vi "PID_2Chan_V3_multiple_avgs.vi"() -> ()   [LabVIEW 2016]
uses:
  <vilib>/addons/control/pid/pid.llb/PID Advanced (DBL Array).vi
  <vilib>/addons/control/pid/pid.llb/PID Parameter Manager (DBL Array).vi
  <vilib>/addons/control/pid/pid.llb/PID Derivative Action Buffered (DBL Array).vi
  <vilib>/addons/control/pid/pid.llb/PID Get Advanced Error (DBL Array).vi
  <vilib>/addons/control/pid/pid.llb/PID Integral Action Buffered (DBL Array).vi
  <vilib>/addons/control/pid/pid.llb/PID Resize 1D Array.vi
  <vilib>/addons/control/pid/pid.llb/PID Get Advanced Error (DBL).vi
  <userlib>/Fluigent/Fluigent MFCS/FluigentMFCS_Full.llb/MFCS_EZ Detect.vi
  <userlib>/Fluigent/Fluigent MFCS/FluigentMFCS_Full.llb/MFCS_EZ Initialization.vi
  <userlib>/Fluigent/Fluigent MFCS/FluigentMFCS_Full.llb/MFCS_EZ Write Channel Pressure.vi
  <userlib>/Fluigent/Fluigent MFCS/FluigentMFCS_Full.llb/MFCS_EZ Close.vi
  <vilib>/addons/control/pid/NI_PID_pid.lvlib
  <vilib>/Analysis/NI_AALBase.lvlib
  <vilib>/Analysis/baseanly.llb/Mean (DBL).vi
panel:
  in  "Vals to display":dbl=400.0
  out "F1 plot":dbl(graph)
  out "F tot":dbl
  in  "F2 PID gains":cluster{"P":dbl, "I":dbl, "D":dbl}={"P"=1.0, "I"=0.01, "D"=0.0} {"D" format="%.3f"; "I" format="%.3f"; "P" format="%.3f"}
  out "F1 Err":T1(graph)
  out "Pressures":dbl[](array[numeric])
  in  "F1 PID gains":cluster{"P":dbl, "I":dbl, "D":dbl}={"P"=1.0, "I"=0.01, "D"=0.0} {"D" format="%.3f"; "I" format="%.3f"; "P" format="%.3f"}
  in  "reinitialize? (F) 2":bool
  out "Flow 1":dbl
  in  "reset Averging":bool
  in  "Set current Pressure\n to manual pressure":bool
  out "Pressures":cluster{"[0]":dbl, "[1]":dbl}(graph)={"[0]"=667.158203125, "[1]"=642.5421752929688}
  out "F0 Err":T1(graph)
  in  "stop":bool=TRUE
  out "F total plot":dbl(graph)
  in  "Valves":enum16{"1", "2", "3", "4", "5", "6", "7", "8"}[](array[ring])=[enum."6", enum."7"]
  in  "Pressure Channels":i16[](array[numeric])=[2, 3]
  in  "Manual Pressure Set":dbl[](array[numeric])=[581.6619074041193, 548.1519459117543]
  in  "PID On":bool=TRUE
  in  "reinitialize? (F)":bool
  in  "Ftot Setpoint":dbl=350.0
  in  "F1 Setpoint":dbl=210.0
  in  "Add Ctrl?":bool
  in  "Boards":enum16{"A", "B", "C"}[](array[ring])=[enum."A", enum."A"]
  in  "Valves":enum16{"1", "2", "3", "4", "5", "6", "7", "8"}[](array[ring])=[enum."5", enum."4"]
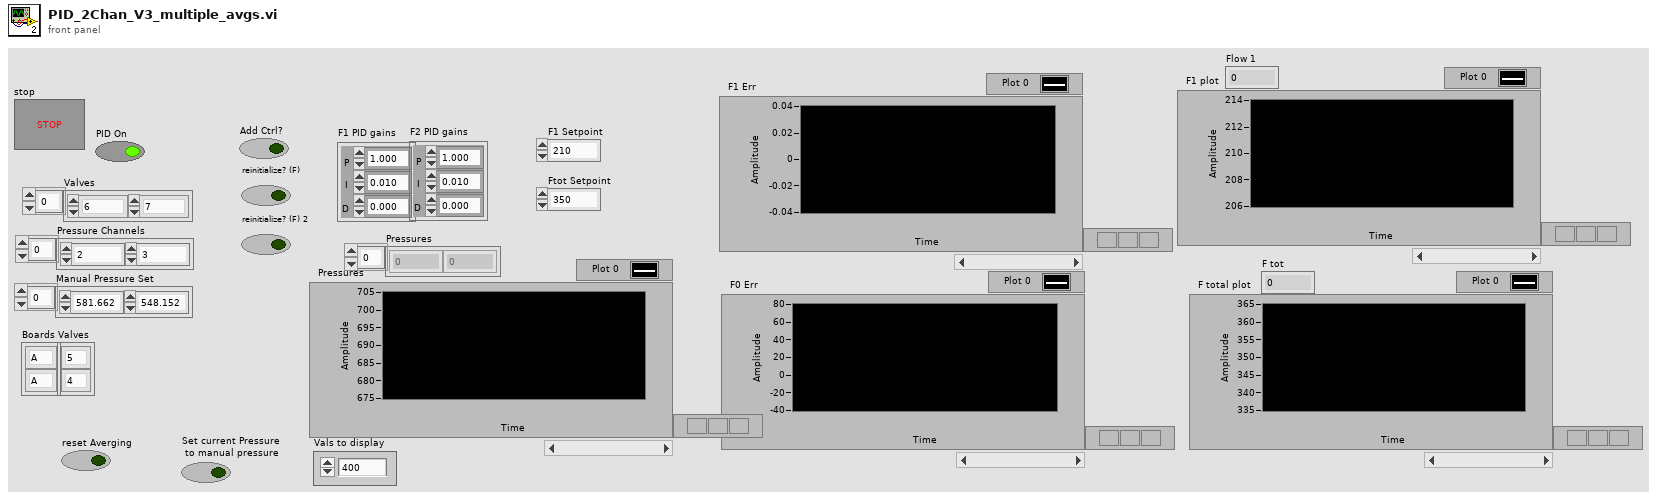
[diagram p1: front panel]
types:
  T1 = cluster{"output[0]":dbl, "output[1]":dbl, "output[2]":dbl}
  T2 = cluster{"setpoint high":dbl, "setpoint low":dbl}[]
  T3 = typedef "_EZmfcsSN.ctl" = u16
  T4 = typedef "_EZmfcsRefNum.ctl" = refnum<k1>
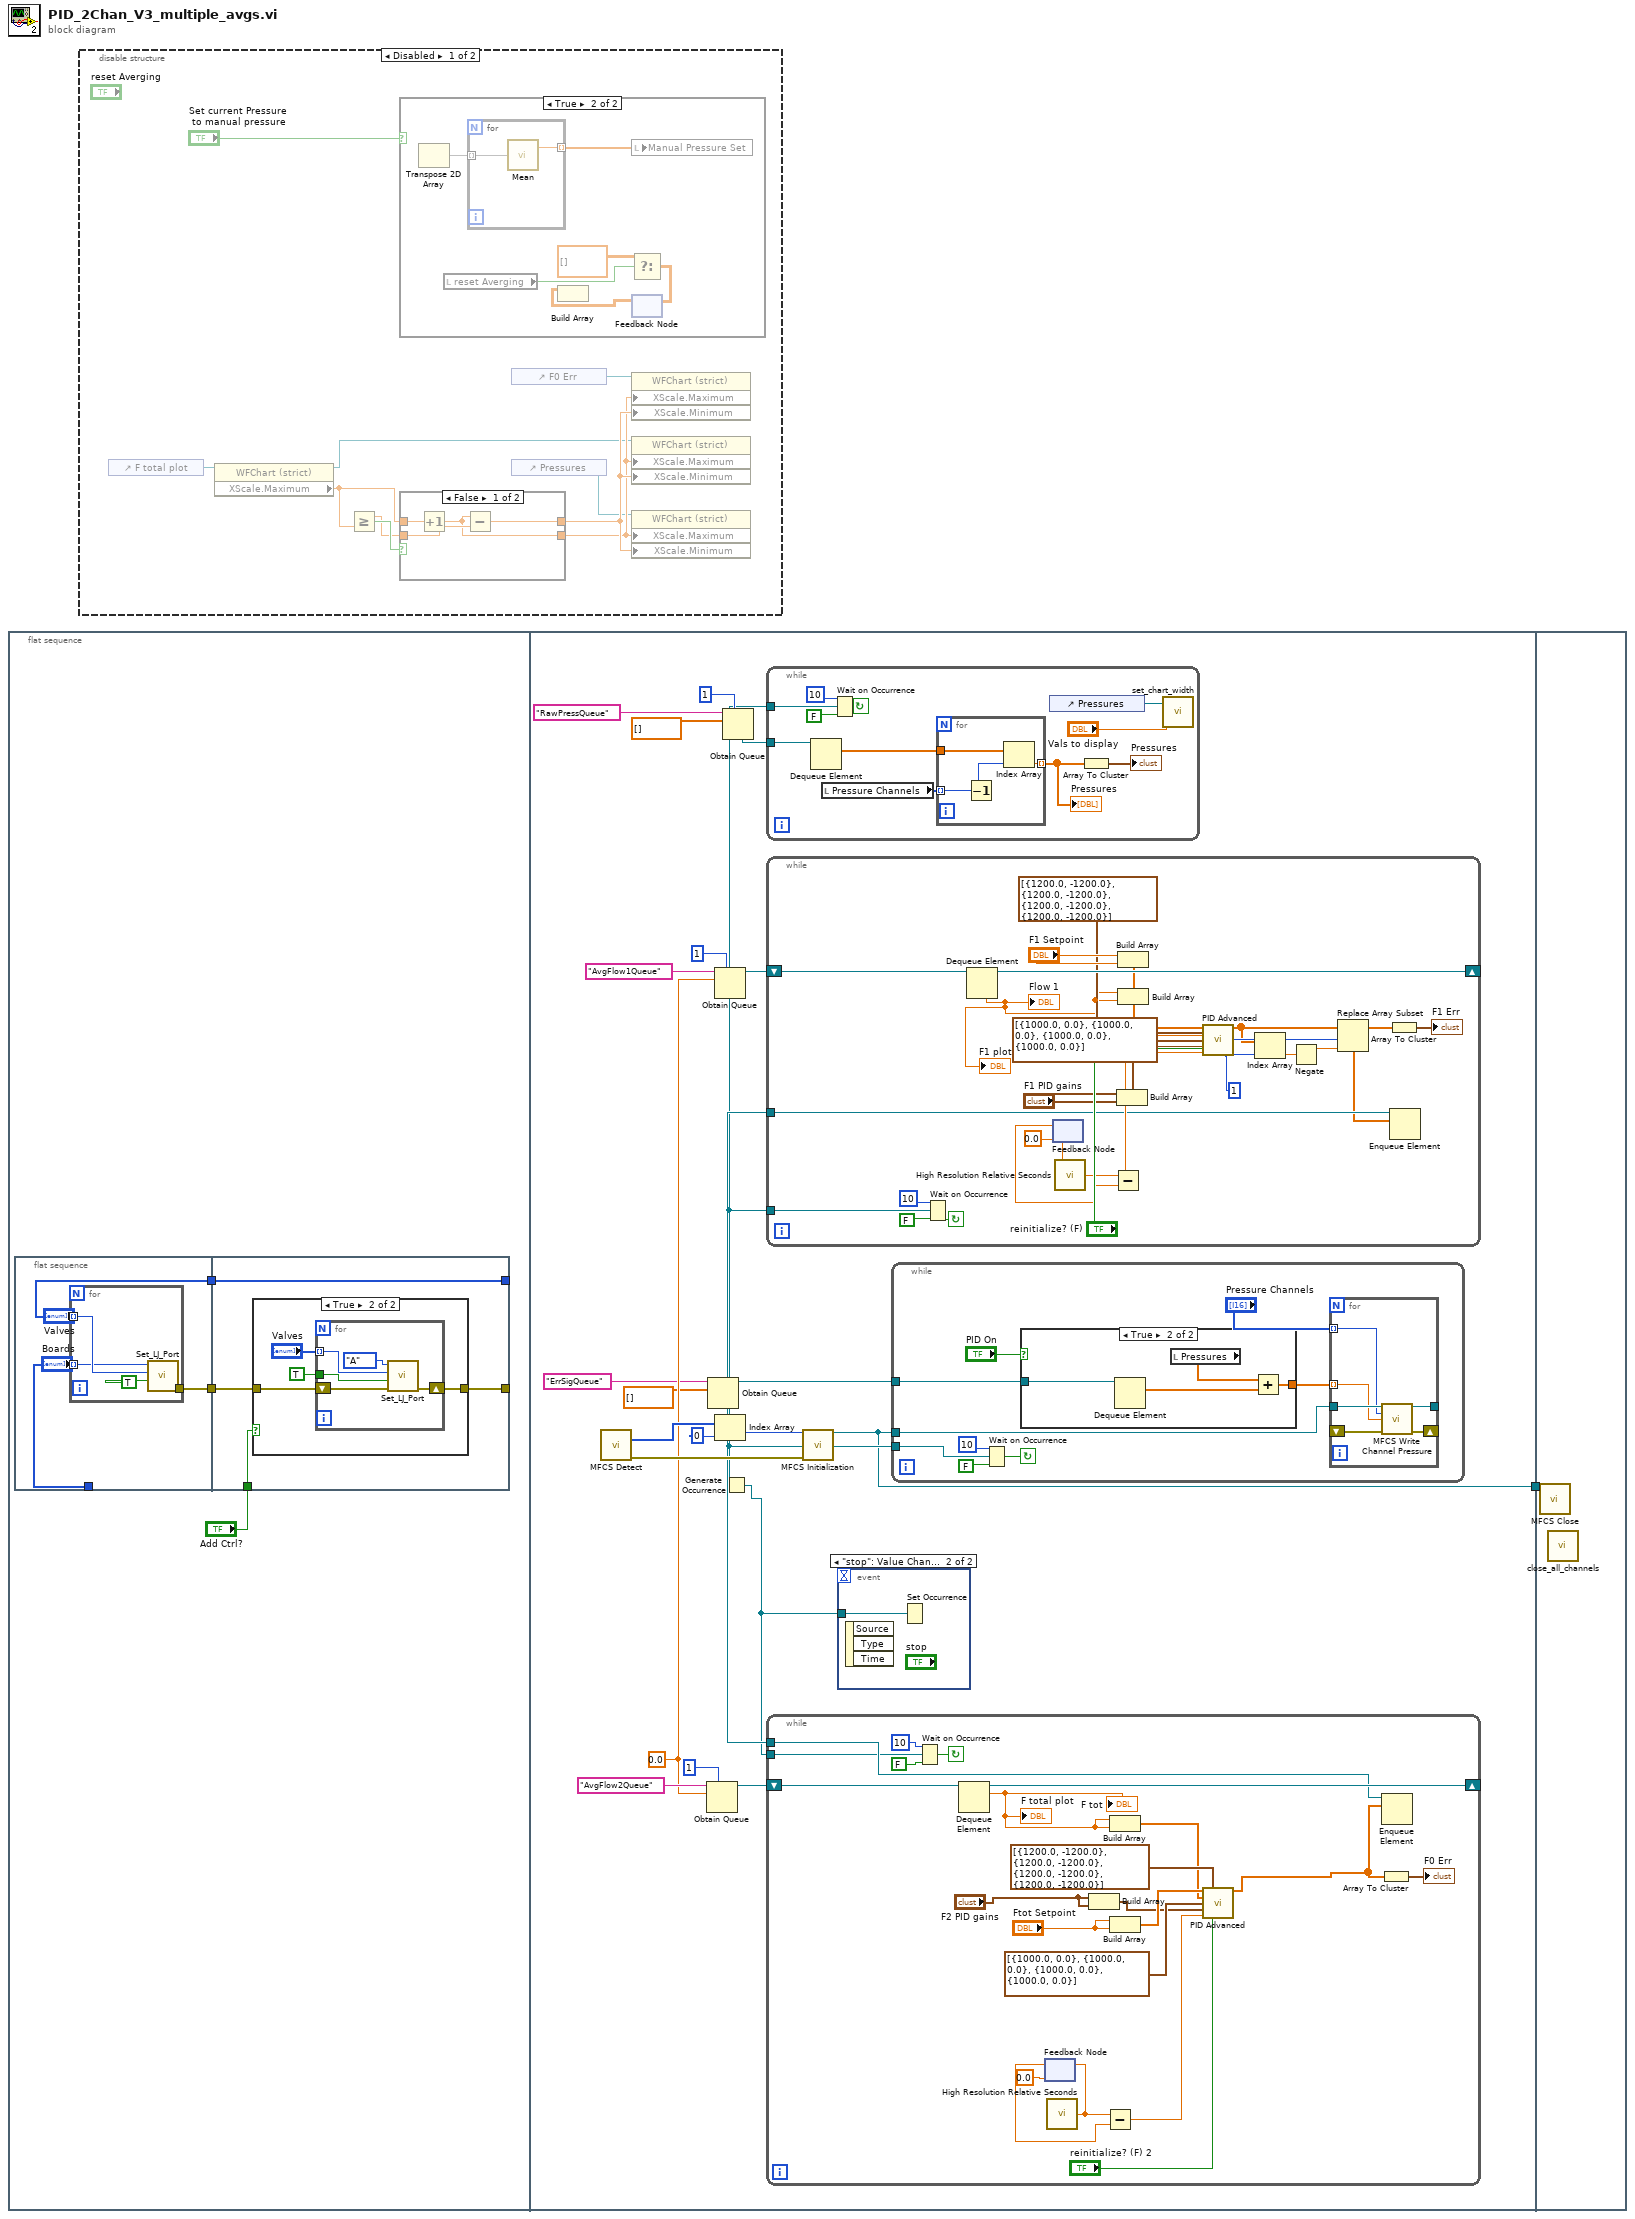
[diagram p0: block diagram]
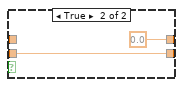
[diagram p2: hidden frame]
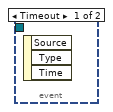
[diagram p6: hidden frame]
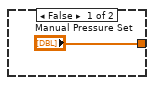
[diagram p7: hidden frame]
diagram:
  n1 = flat-sequence {
    tunnel: [w26] -> w1
    tunnel: w1 -> [w130]
    frame #0 {
      n2 = flat-sequence {
        tunnel: ["Boards"] -> _
        tunnel: [w7] -> w4
        tunnel: ["Valves"] -> w3
        tunnel: [w15] -> _
        tunnel: [w13] -> _
        tunnel: w4 -> [w14]
        tunnel: w3 -> [w15]
        tunnel: "Add Ctrl?" -> [w12]
        frame #0 {
          n3 = for {
            tunnel: "Valves" -> [w11] mode=indexing
            tunnel: "Boards" -> [w10] mode=indexing
            tunnel: [w8] -> w7
            n4 = call "Set_LJ_Port.vi"("State"=TRUE, "Channel"=w11, "Flowboard"=w10) -> ("error out"=w8:errorcluster)  [unwired: 8 in]
          }
        }
        frame #1 {
          n5 = case shown="True" w12 {
            tunnel: w14 -> [w16 w20]
            tunnel: [w16 w19] -> w13
            frame False {
            }
            frame True {
              n6 = for {
                tunnel: TRUE ("State") -> [w23]
                shift-right: [w24] -> w19
                shift-left: w20 -> [w25]
                tunnel: "Valves" -> [w22] mode=indexing
                n7 = call "Set_LJ_Port.vi"("error in"=w25, "State"=w23, "Channel"=w22, "Flowboard"=enum16{"A", "B", "C"}."A") -> ("error out"=w24:errorcluster)  [unwired: 7 in]
              }
            }
          }
        }
      }
    }
    frame #1 {
      w33 = 0.0 ("mean")
      n8 = call-poly <userlib>:"MFCS Detect.vi"() -> ("[SN MFCS_EZ]"=w45:T3[], "error out"=w43:errorcluster)  [unwired: 14 in]
      n9 = Obtain Queue(max queue size (-1, unlimited)=1, name (unnamed)="AvgFlow2Queue", element data type=w33) -> (queue out=w30:refnum<queue>)  [unwired: 2 in, 2 out]
      n10 = Obtain Queue(name (unnamed)="ErrSigQueue", element data type=dbl[] [] ("output array")) -> (queue out=w29:refnum<queue>)  [unwired: 3 in, 2 out]
      n11 = Obtain Queue(max queue size (-1, unlimited)=1, name (unnamed)="AvgFlow1Queue", element data type=w33) -> (queue out=w36:refnum<queue>)  [unwired: 2 in, 2 out]
      n12 = Index Array(array=w45, index=0) -> (element=w44:T3)
      n13 = Generate Occurrence() -> (w27:refnum<k4>)
      n14 = Obtain Queue(max queue size (-1, unlimited)=1, name (unnamed)="RawPressQueue", element data type=dbl[] [] ("appended array")) -> (queue out=w28:refnum<queue>)  [unwired: 2 in, 2 out]
      n15 = while {
        tunnel: w28 -> [w56]
        tunnel: w27 -> [w53]
        stop <- w52 continue-if-true
        n16 = Dequeue Element(queue=w56) -> (element=w50:dbl[])  [unwired: 2 in, 3 out]
        n17 = local read "Pressure Channels"() -> (w51:i16[])
        n18 = Wait on Occurrence(1:FALSE ("ignore previous (T)"), 2:w53, 3:10 ("ms timeout (-1)")) -> (0:w52:bool)
        n19 = for {
          tunnel: w51 -> [w60] mode=indexing
          tunnel: w50 -> [w61]
          tunnel: [w58] -> w49 mode=indexing
          n20 = Decrement(x=w60) -> (x-1=w59:i16)
          n21 = Index Array(array=w61, index=w59) -> (element=w58:dbl)
        }
        "Pressures" <- w49
        n22 = control-ref of="Pressures"() -> (w47:refnum<vi>)
        n23 = Array To Cluster(array=w49) -> (cluster=→"Pressures":cluster{"[0]":dbl, "[1]":dbl})
        n24 = call "set_chart_width.vi"("Values to Display"="Vals to display", "Ref In"=w47) -> ()  [unwired: 10 in]
      }
      n25 = while {
        shift-right: [w128] -> _
        shift-left: w36 -> [w129]
        tunnel: w29 -> [w113]
        tunnel: w27 -> [w108]
        stop <- w107 continue-if-true
        w118 = 1 ("index")
        n26 = Wait on Occurrence(1:FALSE ("ignore previous (T)"), 2:w108, 3:10 ("ms timeout (-1)")) -> (0:w107:bool)
        n27 = Dequeue Element(queue=w129) -> (queue out=w128:refnum<queue>, element=w104:dbl)  [unwired: 2 in, 2 out]
        "Flow 1" <- w104
        "F1 plot" <- w104
        n28 = feedback #1(0.0 ("relative seconds")) -> (w122:dbl)
        n29 = call <vilib>:"High Resolution Relative Seconds.vi"() -> ("relative seconds"=w121:dbl)
        n30 = feedback-in #1(w121) -> ()
        n31 = Subtract(x=w121, y=w122) -> (x-y=w120:dbl)
        n32 = Build Array("F1 PID gains", "F1 PID gains") -> (w111:cluster{"P":dbl, "I":dbl, "D":dbl}[])
        n33 = Build Array("F1 Setpoint", "F1 Setpoint") -> (w126:dbl[])
        n34 = Build Array(w104, w104) -> (w114:dbl[])
        n35 = call-poly <vilib>:"PID Advanced.vi"("setpoint"=w126, "output range"=cluster{"output high":dbl, "output low":dbl}[] [{"output high"=1200.0, "output low"=-1200.0}, {"output high"=1200.0, "output low"=-1200.0}, {"output high"=1200.0, "output low"=-1200.0}, {"output high"=1200.0, "output low"=-1200.0}], "process variable"=w114, "setpoint range"=T2 [{"setpoint high"=1000.0, "setpoint low"=0.0}, {"setpoint high"=1000.0, "setpoint low"=0.0}, {"setpoint high"=1000.0, "setpoint low"=0.0}, {"setpoint high"=1000.0, "setpoint low"=0.0}], "PID gains"=w111, "dt (s)"=w120, "reinitialize? (F)"="reinitialize? (F)") -> ("output"=w115:dbl[])  [unwired: 7 in, 1 out]
        n36 = Index Array(array=w115, index=w118) -> (element=w117:dbl)
        n37 = Negate(x=w117) -> (-x=w116:dbl)
        n38 = Replace Array Subset(array=w115, new element=w116, index=w118) -> (w106:dbl[])
        n39 = Array To Cluster(array=w106) -> (cluster=→"F1 Err":T1)
        n40 = Enqueue Element(queue=w113, element=w106) -> ()  [unwired: 2 in, 3 out]
      }
      n41 = while {
        shift-right: [w102] -> _
        shift-left: w30 -> [w103]
        tunnel: w29 -> [w92]
        tunnel: w27 -> [w90]
        stop <- w87 continue-if-true
        n42 = Wait on Occurrence(1:FALSE ("ignore previous (T)"), 2:w90, 3:10 ("ms timeout (-1)")) -> (0:w87:bool)
        n43 = Dequeue Element(queue=w103) -> (queue out=w102:refnum<queue>, element=w86:dbl)  [unwired: 2 in, 2 out]
        "F total plot" <- w86
        "F tot" <- w86
        n44 = feedback #2(0.0 ("relative seconds")) -> (w97:dbl)
        n45 = call <vilib>:"High Resolution Relative Seconds.vi"() -> ("relative seconds"=w96:dbl)
        n46 = feedback-in #2(w96) -> ()
        n47 = Build Array("F2 PID gains", "F2 PID gains") -> (w83:cluster{"P":dbl, "I":dbl, "D":dbl}[])
        n48 = Subtract(x=w96, y=w97) -> (x-y=w95:dbl)
        n49 = Build Array(w86, w86) -> (w93:dbl[])
        n50 = Build Array("Ftot Setpoint", "Ftot Setpoint") -> (w101:dbl[])
        n51 = call-poly <vilib>:"PID Advanced.vi"("setpoint"=w101, "output range"=cluster{"output high":dbl, "output low":dbl}[] [{"output high"=1200.0, "output low"=-1200.0}, {"output high"=1200.0, "output low"=-1200.0}, {"output high"=1200.0, "output low"=-1200.0}, {"output high"=1200.0, "output low"=-1200.0}], "process variable"=w93, "setpoint range"=T2 [{"setpoint high"=1000.0, "setpoint low"=0.0}, {"setpoint high"=1000.0, "setpoint low"=0.0}, {"setpoint high"=1000.0, "setpoint low"=0.0}, {"setpoint high"=1000.0, "setpoint low"=0.0}], "PID gains"=w83, "dt (s)"=w95, "reinitialize? (F)"="reinitialize? (F) 2") -> ("output"=w82:dbl[])  [unwired: 7 in, 1 out]
        n52 = Array To Cluster(array=w82) -> (cluster=→"F0 Err":T1)
        n53 = Enqueue Element(queue=w92, element=w82) -> ()  [unwired: 2 in, 3 out]
      }
      n54 = call-poly <userlib>:"MFCS Initialization.vi"("SN MFCS_EZ"=w44, "error in (no error)"=w43) -> ("MFCS_EZ"=w26:T4)  [unwired: 11 in, 2 out]
      n55 = event shown="[1] \"stop\": Value Change" {
        selector: _ -> [_ _]
        dyn-events: _ -> [_ _]
        timeout: _ -> [_ _]
        tunnel: w27 -> [_ w46]
        event Timeout {
          n56 = event-data() -> ()  [unwired: 1 in, 3 out]
        }
        event "stop": Value Change {
          n57 = event-data() -> ()  [unwired: 1 in, 3 out]
          n58 = Set Occurrence(w46) -> ()
        }
      }
      n59 = while {
        tunnel: w27 -> [w68]
        tunnel: w29 -> [w66]
        tunnel: w26 -> [w64]
        stop <- w67 continue-if-true
        n60 = Wait on Occurrence(1:FALSE ("ignore previous (T)"), 2:w68, 3:10 ("ms timeout (-1)")) -> (0:w67:bool)
        n61 = case shown="True" "PID On" {
          tunnel: w66 -> [_ w81]
          tunnel: ["Manual Pressure Set" w78] -> w62
          frame False {
          }
          frame True {
            n62 = Dequeue Element(queue=w81) -> (element=w80:dbl[])  [unwired: 2 in, 3 out]
            n63 = local read "Pressures"() -> (w79:dbl[])
            n64 = Add(x=w79, y=w80) -> (x+y=w78:dbl[])
          }
        }
        n65 = for {
          shift-right: [w75] -> _
          shift-left: _ -> [w76]
          tunnel: [w74] -> _
          tunnel: w64 -> [w73]
          tunnel: "Pressure Channels" -> [w72] mode=indexing
          tunnel: w62 -> [w71] mode=indexing
          n66 = call-poly <userlib>:"MFCS Write Channel Pressure.vi"("MFCS_EZ"=w73, "Channel Number (default=1)"=w72, "Pressure (mBar)"=w71, "error in (no error)"=w76) -> ("MFCS_EZ out"=w74:T4, "error out"=w75:errorcluster)  [unwired: 10 in]
        }
      }
    }
    frame #2 {
      n67 = call-poly <userlib>:"MFCS Close.vi"("MFCS_EZ"=w130) -> ()  [unwired: 14 in, 1 out]
      n68 = call "close_all_channels.vi"() -> ()  [unwired: 12 in]
    }
  }
  n69 = disable-structure shown="Disabled" {
    frame Disabled {
      n70 = control-ref of="F total plot"() -> (w134:refnum<vi>)
      n71 = property on="Property Node" class="WFChart (strict)"(reference=w134) -> (reference out=w135:refnum<vi>, "XScale.Maximum"=w133:dbl)  [unwired: 1 in, 1 out]
      n72 = Greater Or Equal?(y=w133) -> (x=w131:dbl, x >= y?=w132:bool)
      n73 = case shown="True" "Set current Pressure\n to manual pressure" {
        frame False {
        }
        frame True {
          n74 = Transpose 2D Array() -> (transposed array=w150:dbl[][])  [unwired: 1 in]
          n75 = local read "reset Averging"() -> (w151:bool)
          n76 = for {
            tunnel: w150 -> [w154] mode=indexing
            tunnel: [w153] -> w147 mode=indexing
            n77 = call-poly <vilib>:"Mean.vi"("X"=w154) -> ("mean"=w153:dbl)  [unwired: 1 out]
          }
          n78 = local write "Manual Pressure Set"(w147) -> ()
          n79 = Select(t=dbl[][] [] ("appended array"), s=w151) -> (s? t:f=w148:dbl[][])  [unwired: 1 in]
          n80 = feedback-in #3(w148) -> ()
          n81 = feedback #3() -> (w152:dbl[][])  [unwired: 1 in]
          n82 = Build Array(w152) -> ()  [unwired: 1 in, 1 out]
        }
      }
      n83 = case shown="False" w132 {
        tunnel: w131 -> [w142 w146]
        tunnel: w133 -> [w144 _]
        tunnel: [w141 w146] -> w138
        tunnel: [w143 0.0] -> w139
        frame False {
          n84 = Increment(x=w144) -> (x+1=w141:dbl)
          n85 = Subtract(x=w141, y=w142) -> (x-y=w143:dbl)
        }
        frame True {
        }
      }
      n86 = control-ref of="F0 Err"() -> (w137:refnum<vi>)
      n87 = control-ref of="Pressures"() -> (w136:refnum<vi>)
      n88 = property on="Property Node" class="WFChart (strict)"(reference=w137, "XScale.Maximum"=w138, "XScale.Minimum"=w139) -> ()  [unwired: 1 in, 2 out]
      n89 = property on="Property Node" class="WFChart (strict)"(reference=w135, "XScale.Maximum"=w138, "XScale.Minimum"=w139) -> ()  [unwired: 1 in, 2 out]
      n90 = property on="Property Node" class="WFChart (strict)"(reference=w136, "XScale.Maximum"=w138, "XScale.Minimum"=w139) -> ()  [unwired: 1 in, 2 out]
    }
    frame Enabled {
    }
  }
